vi "getposy.vi"(11 "shift":dbl) -> (3 "function return":dbl)   [LabVIEW 2017, in "HapticSTM.lvlib"]
doc: "extern \"C\" __declspec(dllexport) double getposy();\nextern \"C\" __declspec(dllexport) double getposy(double shift);"
uses:
  HapticSTM.lvlib
  <userlib>/HapticSTM/HapticSTM.dll
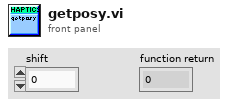
[diagram p1: front panel]
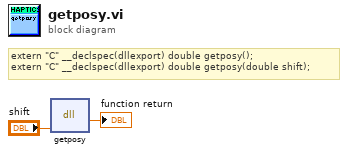
[diagram p0: block diagram]
diagram:
  # "extern \"C\" __declspec(dllexport) double getposy();\nextern \"C\" __declspec(dllexport) double getposy(double shift);"
  n1 = dll-call lib="C:/Program Files/National Instruments/LabVIEW 2019/user.lib/HapticSTM/HapticSTM.*" fn="getposy"("shift"="shift") -> (→"function return":dbl)  [unwired: 4 in, 2 out]
